vi "Prompt for Terminal Counts.vi"() -> (1 "Canceled?":bool, 3 "Terminal Counts":T1)   [LabVIEW 2015]
panel:
  in  "Cancel":bool
  in  "OK":bool
  in  "Path":u32
  in  "String":u32
  in  "Numeric":u32
  # "How many terminals of\neach type are there, including clusters, etc.?"
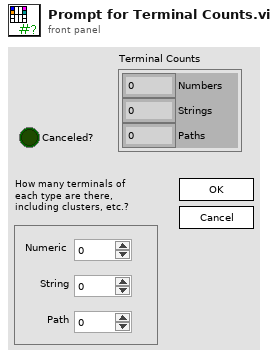
[diagram p1: front panel]
types:
  T1 = cluster{"Numbers":u32, "Strings":u32, "Paths":u32}
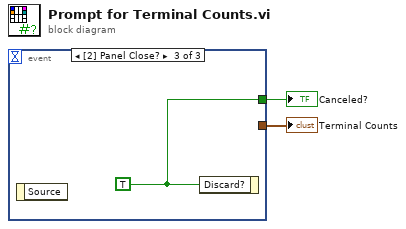
[diagram p0: block diagram]
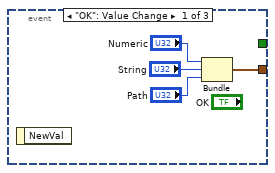
[diagram p2: hidden frame]
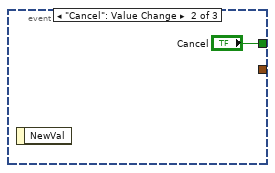
[diagram p3: hidden frame]
diagram:
  n1 = event shown="[2] Panel Close?" {
    selector: _ -> [_ _ _]
    dyn-events: _ -> [_ _ _]
    timeout: _ -> [_ _ _]
    tunnel: [w3 _ _] -> w2
    tunnel: [_ "Cancel" w8] -> w1
    event "OK": Value Change {
      n2 = event-data() -> ()  [unwired: 1 in, 1 out]
      n3 = Bundle("Numeric"="Numeric", "String"="String", "Path"="Path") -> (w3:cluster{"Numeric":u32, "String":u32, "Path":u32})  [unwired: 1 in]
    }
    event "Cancel": Value Change {
      n4 = event-data() -> ()  [unwired: 1 in, 1 out]
    }
    event Panel Close? {
      w8 = TRUE ("Discard?")
      n5 = event-data() -> ()  [unwired: 1 in, 1 out]
      n6 = event-data("Discard?"=w8) -> ()  [unwired: 1 in, 1 out]
    }
  }
  "Terminal Counts" <- w2
  "Canceled?" <- w1
